vi "Write Scanners.vi"(8 "error in (no error)":errorcluster, 9 "Scanner 2 in":refnum<class "Scanner.lvclass">, 10 "Scanner 1 in":refnum<class "Scanner.lvclass">, 11 "Double Scanner in":refnum<class "Double Scanner.lvclass">) -> (0 "error out":errorcluster, 3 "Double Scanner out":refnum<class "Double Scanner.lvclass">)   [LabVIEW 2023, in "Double Scanner.lvclass"]
uses:
  Double Scanner.lvclass
  Scanner/Scanner.lvclass
  Double Scanner.lvclass/Double Scanner.ctl
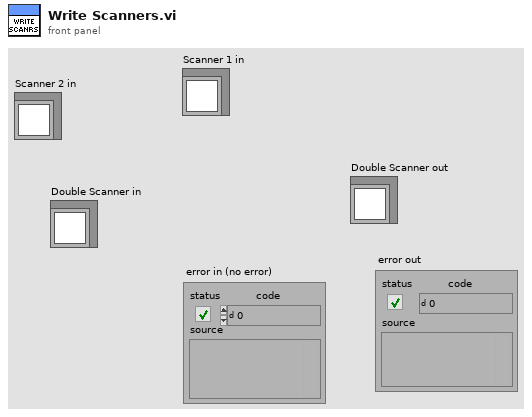
[diagram p1: front panel]
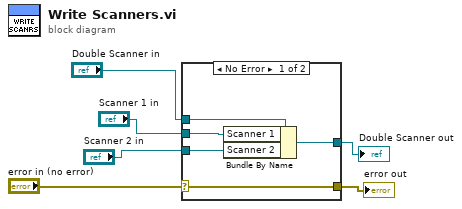
[diagram p0: block diagram]
diagram:
  n1 = case shown="No Error" "error in (no error)" {
    selector: "error in (no error)" -> [w7 w13]
    tunnel: "Scanner 1 in" -> [w11 _]
    tunnel: "Scanner 2 in" -> [w10 _]
    tunnel: "Double Scanner in" -> [w9 w12]
    tunnel: [w8 w12] -> w2
    tunnel: [w7 w13] -> w1
    frame No Error {
      n2 = Bundle By Name(cluster=w9, "Scanner 1"=w11, "Scanner 2"=w10) -> (w8:refnum<class "Double Scanner.lvclass">)
    }
    frame Error {
    }
  }
  "Double Scanner out" <- w2
  "error out" <- w1
